vi "Stop Impl.vi"(11 "Newport Power Meter in":refnum<class "Newport Power Meter.lvclass">) -> (3 "Newport Power Meter out":refnum<class "Newport Power Meter.lvclass">)   [LabVIEW 2023, in "Newport Power Meter.lvlib" / "Newport Power Meter.lvclass"]
uses:
  Newport Power Meter.lvclass
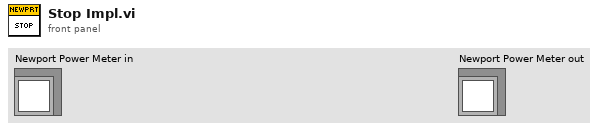
[diagram p1: front panel]
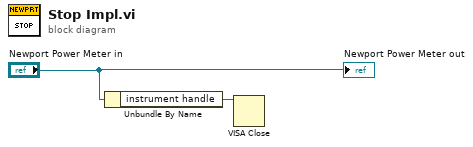
[diagram p0: block diagram]
diagram:
  n1 = Unbundle By Name("Newport Power Meter in") -> ("instrument handle"=w2:refnum<visa-resource-name>)
  n2 = VISA Close(VISA resource name=w2) -> ()  [unwired: 1 in, 1 out]
  "Newport Power Meter out" <- "Newport Power Meter in"
